vi "GoalCenter.vi"(8 "CurrentGoalCenterY":dbl, 9 "CurrentGoalCenterX":dbl, 10 "CenterPixelY":dbl, 11 "CenterPixelX":dbl) -> (1 "PsuedoJoystickOutRotation":dbl)   [LabVIEW 2012]
panel:
  # "Inputs"
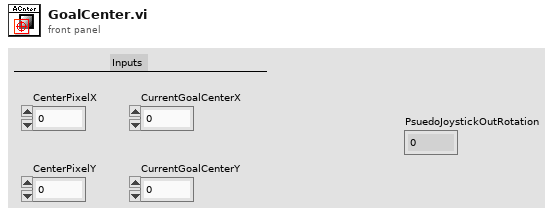
[diagram p1: front panel]
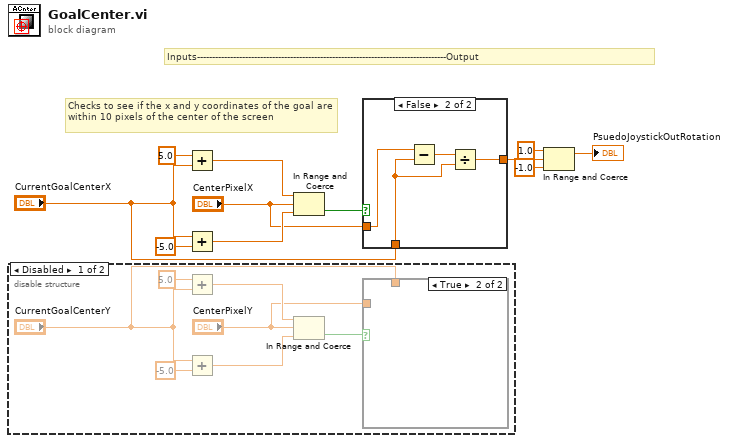
[diagram p0: block diagram]
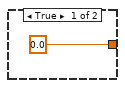
[diagram p4: hidden frame]
diagram:
  # "Inputs-----------------------------------------------------------------------------------Output"
  # "Checks to see if the x and y coordinates of the goal are within 10 pixels of the center of the screen"
  n1 = disable-structure shown="Disabled" {
    frame Disabled {
      n2 = Add(x=5.0, y="CurrentGoalCenterY") -> (x+y=w18:dbl)
      n3 = Add(x="CurrentGoalCenterY", y=-5.0) -> (x+y=w15:dbl)
      n4 = In Range and Coerce(upper limit=w18, x="CenterPixelY", lower limit=w15) -> (In Range?=w14:bool)  [unwired: 1 out]
      n5 = case shown="True" w14 {
        tunnel: "CurrentGoalCenterY" -> [_ _]
        tunnel: "CenterPixelY" -> [_ _]
        frame False {
        }
        frame True {
        }
      }
    }
    frame Enabled {
    }
  }
  n6 = Add(x=5.0, y="CurrentGoalCenterX") -> (x+y=w11:dbl)
  n7 = Add(x="CurrentGoalCenterX", y=-5.0) -> (x+y=w8:dbl)
  n8 = In Range and Coerce(upper limit=w11, x="CenterPixelX", lower limit=w8) -> (In Range?=w7:bool)  [unwired: 1 out]
  n9 = case shown="False" w7 {
    tunnel: "CurrentGoalCenterX" -> [_ w20]
    tunnel: "CenterPixelX" -> [_ w23]
    tunnel: [0.0 w21] -> w3
    frame True {
    }
    frame False {
      n10 = Subtract(x=w23, y=w20) -> (x-y=w22:dbl)
      n11 = Divide(x=w22, y=w20) -> (x/y=w21:dbl)
    }
  }
  n12 = In Range and Coerce(upper limit=1.0, x=w3, lower limit=-1.0) -> (coerced(x)=→"PsuedoJoystickOutRotation":dbl)  [unwired: 1 out]
